vi "ParGetLastError.vi"(0 "ref in":u64, 11 "error in (no error)":errorcluster) -> (4 "ref out":u64, 6 "Result":i32, 8 "LastError":i32, 15 "error out":errorcluster)   [LabVIEW 2020, in "Snap7.lvlib"]
uses:
  Snap7.lvlib
  windows/lv_snap7.dll
panel:
  in  "var lasterror":i32
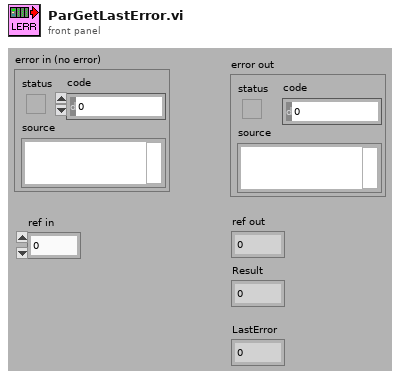
[diagram p1: front panel]
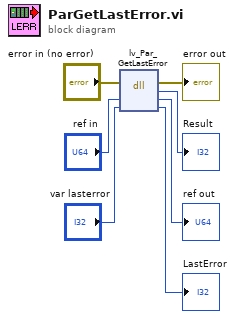
[diagram p0: block diagram]
diagram:
  n1 = dll-call lib="PTH2iabs CUsersFeng项目HLCEPS300-1老性能试验台SourcesSnap7libwindowslv_snap7.dll" fn="lv_Par_GetLastError"(error in="error in (no error)", "Partner"="ref in", "LastError"="var lasterror") -> (error out=→"error out":errorcluster, "return type"=→"Result":i32, "Partner"=→"ref out":u64, "LastError"=→"LastError":i32)  [unwired: 2 in, 1 out]
